vi "Get VI Path.vi"(8 "error in (no error)":errorcluster, 11 "VI Reference":refnum<vi>) -> (0 "error out":errorcluster, 2 "VI Path":path, 3 "reference out":refnum<vi>)   [LabVIEW 2010]
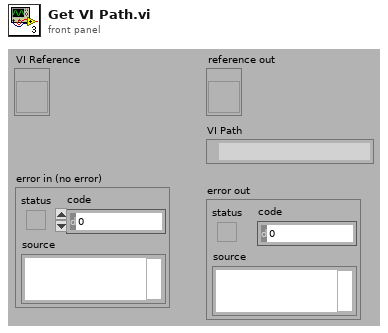
[diagram p1: front panel]
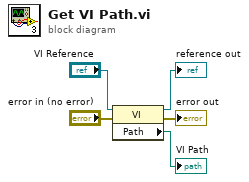
[diagram p0: block diagram]
diagram:
  n1 = property class="VI"(reference="VI Reference", error in="error in (no error)") -> (reference out=→"reference out":refnum<vi>, error out=→"error out":errorcluster, "Path"=→"VI Path":path)
